vi "Destroy Queues.vi"(8 "error in (no error)":errorcluster) -> (0 "error out":errorcluster)   [LabVIEW 2016, in "System.lvlib"]
uses:
  System.lvlib
  Controls/Control_Queue Reference.ctl
  Controls/Control_Message Data.ctl
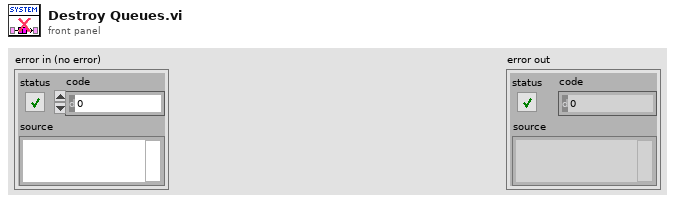
[diagram p1: front panel]
types:
  T1 = typedef "System.lvlib/Control_Variant Data Reference.ctl" = refnum<data-value>
  T2 = typedef "System.lvlib/Control_Queue Reference.ctl" = refnum<queue>
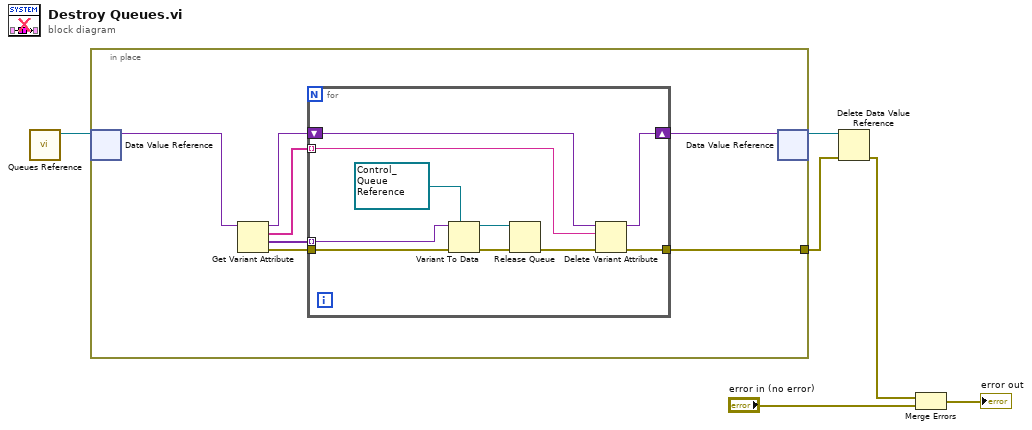
[diagram p0: block diagram]
diagram:
  n1 = call "Queues Reference.vi"() -> ("Queues Reference"=w6:T1)  [unwired: 10 in, 1 out]
  n2 = in-place {
    in-place-border: [w13] -> w4
    n3 = in-place-dvr #1(w6) -> (w8:variant)  [unwired: 1 out]
    n4 = Get Variant Attribute(Variant=w8) -> (duplicate Variant=w10:variant, names=w9:string[], values=w11:variant[], error out=w12:errorcluster)  [unwired: 3 in]
    n5 = for {
      tunnel: w12 -> [w23]
      tunnel: w11 -> [w22] mode=indexing
      shift-right: [w19] -> w7
      shift-left: w10 -> [w17]
      tunnel: w9 -> [w16] mode=indexing
      tunnel: [w15] -> w13
      n6 = Variant To Data(error in=w23, type=T2 refnum ("queue"), Variant=w22) -> (data=w20:T2, error out=w21:errorcluster)
      n7 = Release Queue(queue=w20, error in (no error)=w21) -> (error out=w18:errorcluster)  [unwired: 1 in, 2 out]
      n8 = Delete Variant Attribute(4:w18, 6:w16, 7:w17) -> (0:w15:errorcluster, 3:w19:variant)  [unwired: 1 out]
    }
    n9 = in-place-dvr #1(w7) -> (w5:T1)  [unwired: 1 out]
  }
  n10 = Delete Data Value Reference(data value reference=w5, error in=w4) -> (error out=w3:errorcluster)  [unwired: 1 out]
  n11 = Merge Errors(w3, "error in (no error)") -> (→"error out":errorcluster)
